vi "10_to_256.vi"(1 "Decimal":dbl format="%#_13g") -> (0 "256":u8[](array[numeric]))   [LabVIEW 2015, in "Igor.lvclass"]
uses:
  Igor.lvclass
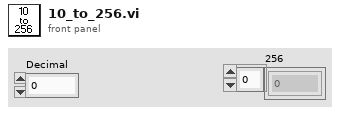
[diagram p1: front panel]
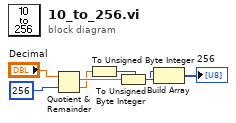
[diagram p0: block diagram]
diagram:
  n1 = Quotient & Remainder(x="Decimal", y=256) -> (x-y*floor(x/y)=w5:dbl, floor(x/y)=w4:dbl)
  n2 = To Unsigned Byte Integer(number=w4) -> (unsigned 8bit integer=w3:u8)
  n3 = To Unsigned Byte Integer(number=w5) -> (unsigned 8bit integer=w2:u8)
  n4 = Build Array(w2, w3) -> (→"256":u8[])
